vi "Load Programs.vi"(0 "Program List in":refnum<class "Program List From SFTP.lvclass">, 5 "error in (no error)":errorcluster, 8 "Application.lvclass":refnum<class "Application.lvclass">) -> (14 "Program List out":refnum<class "Program List From SFTP.lvclass">, 15 "Programs":string[](array[string]), 19 "error out":errorcluster)   [LabVIEW 2019, in "Program List From SFTP.lvclass"]
uses:
  Program List From SFTP.lvclass
  Application.lvclass
  Program List From SFTP.lvclass/Program List From SFTP.ctl
  LabSSH Library/SFTP Library/LabSFTP.lvlib
panel:
  out "Script Files":string[](array[string])
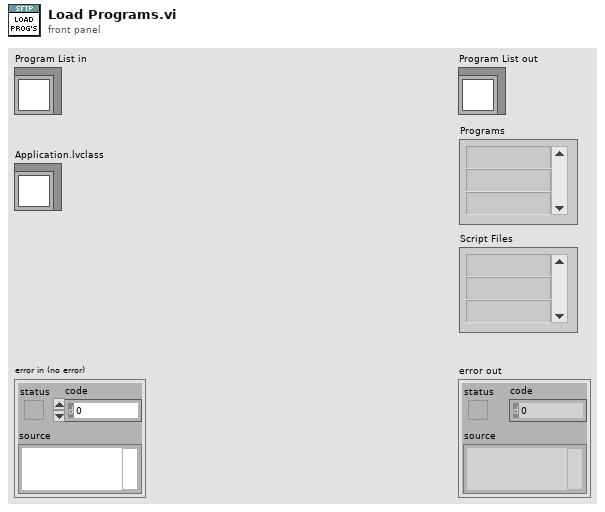
[diagram p1: front panel]
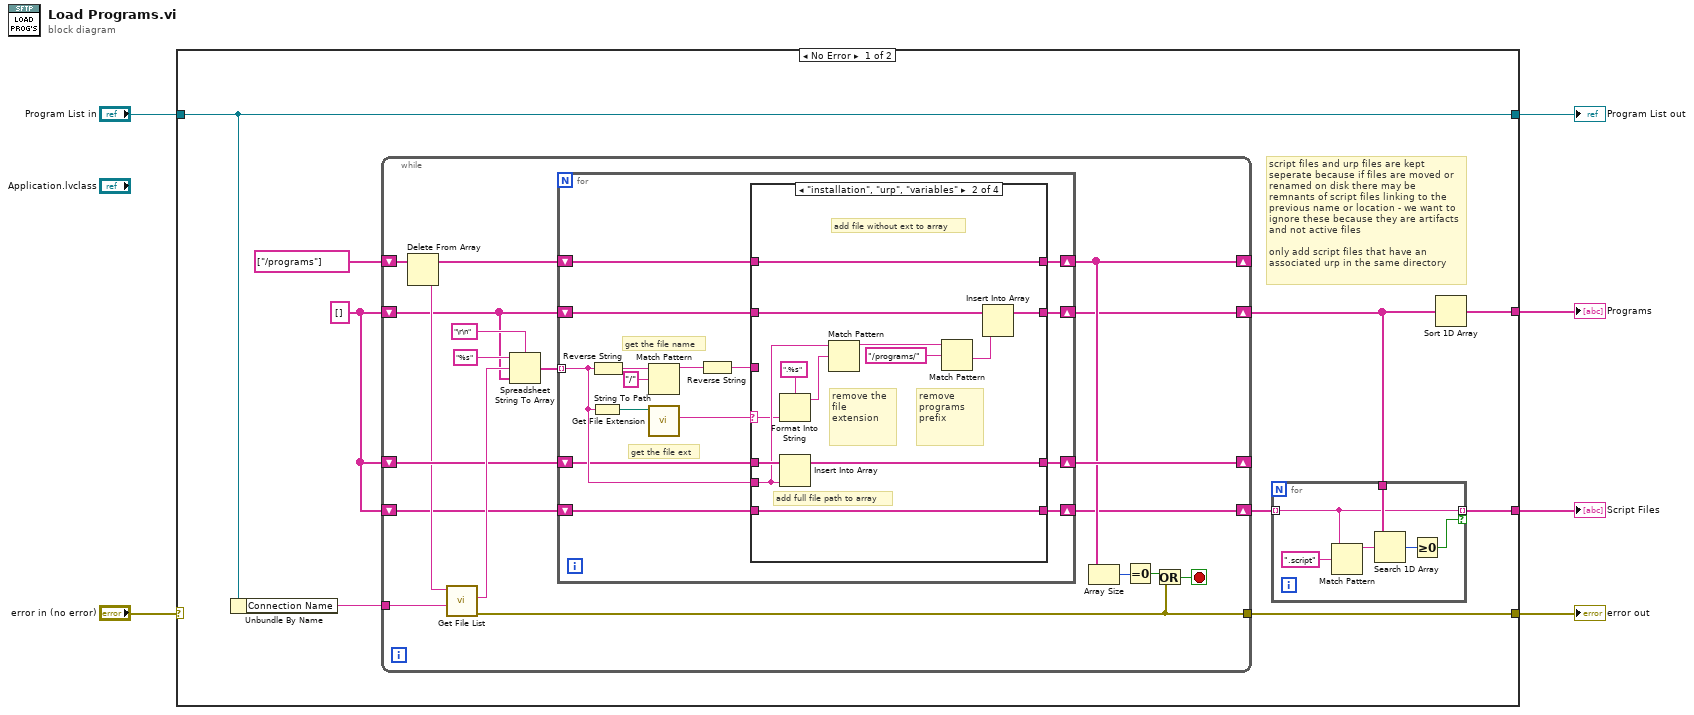
[diagram p0: block diagram]
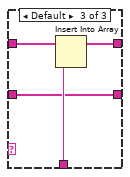
[diagram p4: hidden frame]
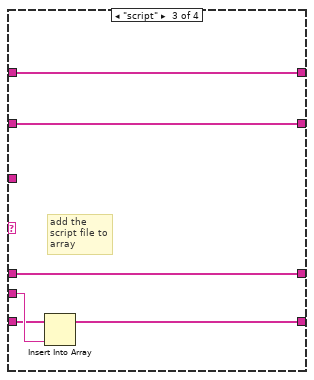
[diagram p5: hidden frame]
diagram:
  n1 = case shown="No Error" "error in (no error)" {
    selector: "error in (no error)" -> [_ w96]
    tunnel: [w8 _] -> w6
    tunnel: [w12 _] -> w5
    tunnel: [w11 w96] -> w4
    tunnel: "Program List in" -> [w9 w95]
    tunnel: [w9 w95] -> w1
    frame No Error {
      w13 = string[] []
      # "script files and urp files are kept seperate because if files are moved or renamed on disk there may be remnants of script files linking to the previous name or location - we want to ignore these because they are artifacts and not active files\n\nonly add script files that have an associated urp in the same directory"
      n2 = Unbundle By Name(w9) -> ("Connection Name"=w10:string)
      n3 = while {
        shift-right: [w36] -> _
        shift-left: w13 -> [w35]
        shift-right: [w31] -> _
        shift-left: string[] ["/programs"] -> [w34]
        tunnel: [w28] -> w11
        shift-right: [w26] -> w14
        shift-left: w13 -> [w25]
        shift-right: [w24] -> w7
        shift-left: w13 -> [w23]
        tunnel: w10 -> [w22]
        stop <- w27 stop-if-true
        n4 = Delete From Array(array=w34) -> (deleted portion=w32:string, array with subset deleted=w33:string[])  [unwired: 2 in]
        n5 = call "Get File List.vi"("Connection Name"=w22, "Remote Path"=w32) -> ("error out"=w28:errorcluster, "File List"=w40:string)  [unwired: 7 in, 1 out]
        n6 = Spreadsheet String To Array(delimiter (Tab)="\r\n", format string="%s", spreadsheet string=w40, array type (2D Dbl)=w23) -> (array=w37:string[])
        n7 = for {
          tunnel: w37 -> [w49] mode=indexing
          shift-right: [w48] -> w36
          shift-left: w35 -> [w47]
          shift-right: [w46] -> w31
          shift-left: w33 -> [w45]
          shift-right: [w44] -> w26
          shift-left: w25 -> [w43]
          shift-right: [w42] -> w24
          shift-left: w23 -> [w41]
          # "get the file ext"
          # "get the file name"
          n8 = String To Path(string=w49) -> (path=w53:path)
          n9 = Reverse String(1:w49) -> (0:w55:string)
          n10 = Match Pattern(string=w55, regular expression="/") -> (before substring=w52:string)  [unwired: 1 in, 3 out]
          n11 = call <vilib>:"Get File Extension.vi"("file"=w53) -> ("lowercase file extension"=w51:string)  [unwired: 6 in, 4 out]
          n12 = Reverse String(1:w52) -> (0:w50:string)
          n13 = case shown="\"installation\", \"urp\", \"variables\"" w51 {
            selector: w51 -> [_ w77 _ _]
            tunnel: w50 -> [w62 _ _ _]
            tunnel: w49 -> [w61 w78 w90 _]
            tunnel: [w63 w84 w88 w94] -> w48
            tunnel: w47 -> [w63 w83 w88 w94]
            tunnel: [w60 w82 w89 w93] -> w46
            tunnel: w45 -> [w59 w82 w89 w93]
            tunnel: [w58 w81 w87 w92] -> w44
            tunnel: w43 -> [w58 w81 w86 w92]
            tunnel: [w56 w80 w85 w91] -> w42
            tunnel: w41 -> [w57 w79 w85 w91]
            frame "" {
              n14 = case shown="\"\", \".\", \"..\"" w62 {
                tunnel: w61 -> [_ _ w71]
                tunnel: [w65 w67 w70] -> w60
                tunnel: w59 -> [w65 w67 w69]
                tunnel: w57 -> [w64 w66 w68]
                tunnel: [w64 w66 w68] -> w56
                frame "", ".", ".." {
                  # "invalid folder"
                }
                frame "usbdisk".."usbdisk~" {
                  # "invalid folder"
                }
                frame Default {
                  n15 = Insert Into Array(array=w69, new element=w71) -> (w70:string[])  [unwired: 1 in]
                }
              }
            }
            frame "installation", "urp", "variables" {
              # "remove programs prefix"
              # "remove the file extension"
              # "add file without ext to array"
              # "add full file path to array"
              n16 = Format Into String(format string=".%s", w77) -> (resulting string=w76:string)  [unwired: 2 in, 1 out]
              n17 = Insert Into Array(array=w83, new element=w78) -> (w84:string[])  [unwired: 1 in]
              n18 = Match Pattern(string=w78, regular expression=w76) -> (before substring=w74:string)  [unwired: 1 in, 3 out]
              n19 = Match Pattern(string=w74, regular expression="/programs/") -> (after substring=w72:string)  [unwired: 1 in, 3 out]
              n20 = Insert Into Array(array=w79, new element=w72) -> (w80:string[])  [unwired: 1 in]
            }
            frame "script" {
              # "add the script file to array"
              n21 = Insert Into Array(array=w86, new element=w90) -> (w87:string[])  [unwired: 1 in]
            }
            frame Default {
            }
          }
        }
        n22 = Array Size(array=w31) -> (size(s)=w30:i32)
        n23 = Equal To 0?(x=w30) -> (x = 0?=w29:bool)
        n24 = Or(x=w29, y=w28) -> (x .or. y?=w27:bool)
      }
      n25 = for {
        tunnel: w14 -> [w18] mode=indexing
        tunnel: [w18] -> w12 mode=indexing if=w19
        tunnel: w7 -> [w21]
        n26 = Match Pattern(string=w18, regular expression=".script") -> (before substring=w16:string)  [unwired: 1 in, 3 out]
        n27 = Search 1D Array(1D array=w21, element=w16) -> (index of element=w20:i32)  [unwired: 1 in]
        n28 = Greater Or Equal To 0?(x=w20) -> (x >= 0?=w19:bool)
      }
      n29 = Sort 1D Array(array=w7) -> (sorted array=w8:string[])
    }
    frame Error {
    }
  }
  "error out" <- w4
  "Program List out" <- w1
  "Programs" <- w6
  "Script Files" <- w5
